vi "OpenVeriStandProjectExplorer.vi"(8 "error in (no error)":errorcluster) -> (0 "error out":errorcluster)   [LabVIEW 2027, in "VeriStandTestUtilities.lvlib"]
uses:
  VeriStandTestUtilities.lvlib
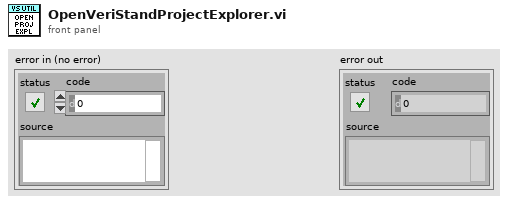
[diagram p1: front panel]
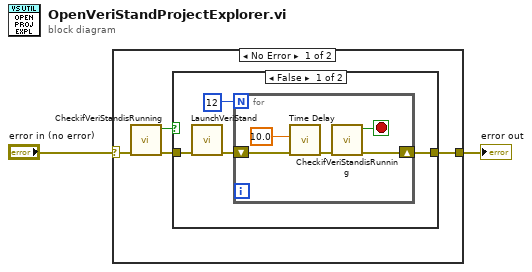
[diagram p0: block diagram]
diagram:
  n1 = case shown="No Error" "error in (no error)" {
    selector: "error in (no error)" -> [w6 w17]
    tunnel: [w5 w17] -> w2
    frame No Error {
      n2 = call "CheckifVeriStandisRunning.vi"("error in (no error)"=w6) -> ("error out"=w4:errorcluster, "VeriStand Running"=w3:bool)  [unwired: 9 in]
      n3 = case shown="False" w3 {
        tunnel: [w9 w16] -> w5
        tunnel: w4 -> [w8 w16]
        frame False {
          n4 = call "LaunchVeriStand.vi"("error in (no error)"=w8) -> ("error out"=w7:errorcluster)  [unwired: 10 in]
          n5 = for {
            N: 12 -> [_]
            shift-right: [w12] -> w9
            shift-left: w7 -> [w14]
            stop <- w11 stop-if-true
            n6 = call "Time Delay"("error in (no error)"=w14, "Delay Time (s)"=10.0) -> ("error out"=w13:errorcluster)  [unwired: 9 in]
            n7 = call "CheckifVeriStandisRunning.vi"("error in (no error)"=w13) -> ("error out"=w12:errorcluster, "VeriStand Running"=w11:bool)  [unwired: 9 in]
          }
        }
        frame True {
        }
      }
    }
    frame Error {
    }
  }
  "error out" <- w2
